vi "call on write tree.vi"(8 "error in":errorcluster, 11 "root":T1) -> (0 "error out":errorcluster)   [LabVIEW 2013, in "NISE_CEF_HierarchyRepo.lvclass"]
uses:
  NISE_CEF_HierarchyRepo.lvclass
  Node/NodeRef.ctl
  Node/NISE_CEF_Node.lvclass
  Node/NISE_CEF_Node.lvclass/NISE_CEF_Node.ctl
  Node/ReadChildren.vi
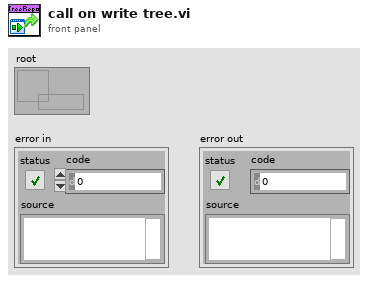
[diagram p1: front panel]
types:
  T1 = typedef "NISE_CEF_Node.lvclass/NodeRef.ctl" = refnum<data-value>
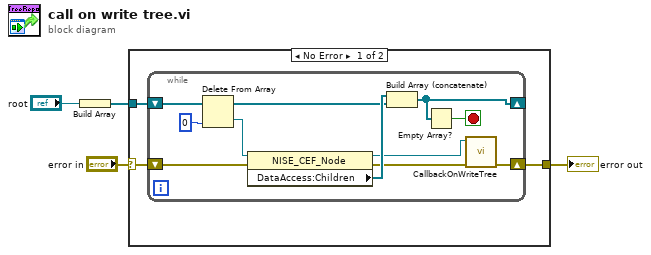
[diagram p0: block diagram]
diagram:
  n1 = Build Array("root") -> (w4:T1[])
  n2 = case shown="No Error" "error in" {
    selector: "error in" -> [w7 w19]
    tunnel: [w6 w19] -> w2
    tunnel: w4 -> [w5 _]
    frame No Error {
      n3 = while {
        shift-right: [w8] -> w6
        shift-left: w7 -> [w16]
        shift-right: [w12] -> _
        shift-left: w5 -> [w18]
        stop <- w11 stop-if-true
        n4 = Delete From Array(array=w18, index=0) -> (deleted portion=w15:T1, array with subset deleted=w13:T1[])  [unwired: 1 in]
        n5 = property class="NISE_CEF_Node"(reference=w15, error in=w16) -> (reference out=w10:T1, error out=w9:errorcluster, "DataAccess:Children"=w14:T1[])
        n6 = Build Array (concatenate)(w14, w13) -> (w12:T1[])
        n7 = Empty Array?(array=w12) -> (empty?=w11:bool)
        n8 = call "CallbackOnWriteTree.vi"("error in"=w9, "node"=w10) -> ("error out"=w8:errorcluster)  [unwired: 9 in]
      }
    }
    frame Error {
    }
  }
  "error out" <- w2
